vi "Reentrancy String.vi"(7 "Format Options":T1={"Background"={"Public Scope"={"Option"=FALSE, "Color"=0, "Operator"=FALSE}, "Protected Scope"={"Option"=FALSE, "Color"=0, "Operator"=FALSE}, "Community Scope"={"Option"=FALSE, "Color"=0, "Operator"=FALSE}, "Private Scope"={"Option"=FALSE, "Color"=0, "Operator"=FALSE}, "Unknown Scope"={"Option"=FALSE, "Color"=0, "Operator"=FALSE}, "Auto Error Handling"={"Option"=FALSE, "Color"=0, "Operator"=FALSE}, "Inline"={"Option"=FALSE, "Color"=0, "Operator"=FALSE}, "Separate CC"={"Option"=FALSE, "Color"=0, "Operator"=FALSE}, "Execution Priority Normal"={"Option"=FALSE, "Color"=0, "Operator"=FALSE}, "Reentrancy Non-RE"={"Option"=FALSE, "Color"=0, "Operator"=FALSE}}, "Bookmark Options"={"Bookmarks as New Line in VI Descriptions"=TRUE, "Unique Bookmark Tags Only"=TRUE, "Include Tag and Text"=TRUE}}, 9 "Exec.IsReentrant":bool, 11 "Exec.ReentrancyType":T4(ring)) -> (1 "Cell Color":u32, 3 "Reentrancy":string)   [LabVIEW 2023, in "VIDoc Printer.lvlib" / "VIDoc Printer.lvclass"]
doc: "Formats Reentrancy information into a string.\nAlso outputs a color based on the Format Options."
uses:
  VIDoc Printer.lvclass
  Settings/Printer Settings/Formatting Options.ctl
  Settings/Printer Settings/Background Formatting Cluster.ctl
  Settings/Printer Settings/Bookmark Options.ctl
  VIDoc Printer.lvclass/VIDoc Printer.ctl
  Settings/Printer Settings/Printer Settings.lvclass
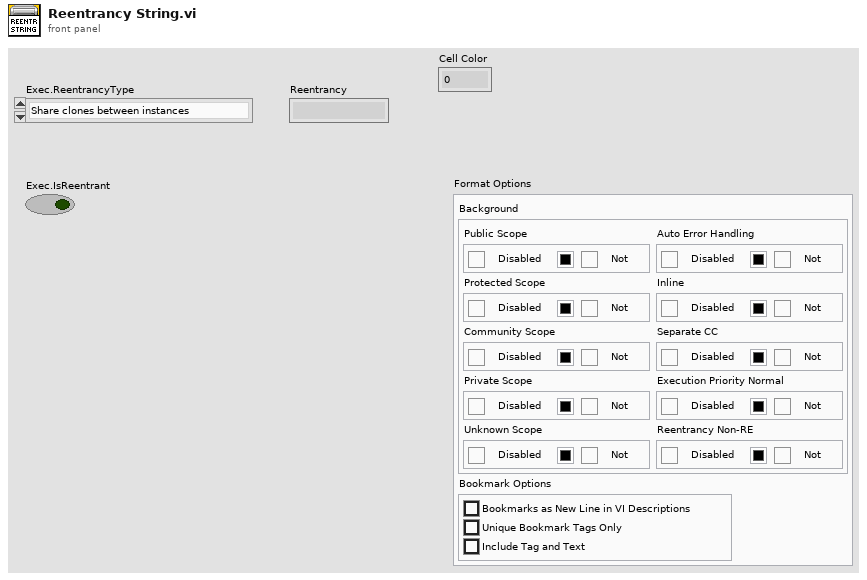
[diagram p1: front panel]
types:
  T1 = typedef "VIDoc Printer.lvlib/Printer Settings.lvclass/Formatting Options.ctl" = cluster{"Background":cluster{"Public Scope":T2, "Protected Scope":T2, "Community Scope":T2, "Private Scope":T2, "Unknown Scope":T2, "Auto Error Handling":T2, "Inline":T2, "Separate CC":T2, "Execution Priority Normal":T2, "Reentrancy Non-RE":T2}, "Bookmark Options":T3}
  T2 = typedef "VIDoc Printer.lvlib/Printer Settings.lvclass/Background Formatting Cluster.ctl" = cluster{"Option":bool, "Color":u32, "Operator":bool}
  T3 = typedef "VIDoc Printer.lvlib/Printer Settings.lvclass/Bookmark Options.ctl" = cluster{"Bookmarks as New Line in VI Descriptions":bool, "Unique Bookmark Tags Only":bool, "Include Tag and Text":bool}
  T4 = enum16{"Share clones between instances", "Preallocate clone for each instance"}
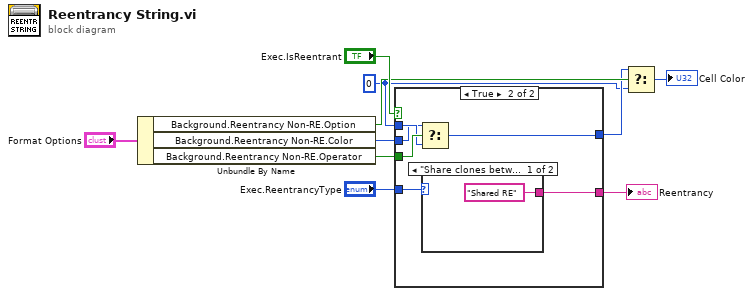
[diagram p0: block diagram]
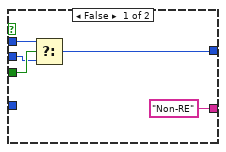
[diagram p2: hidden frame]
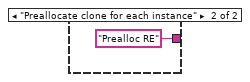
[diagram p3: hidden frame]
diagram:
  w2 = 0
  n1 = Unbundle By Name("Format Options") -> ("Background.Reentrancy Non-RE.Option"=w7:bool, "Background.Reentrancy Non-RE.Color"=w6:u32, "Background.Reentrancy Non-RE.Operator"=w4:bool)
  n2 = case shown="True" "Exec.IsReentrant" {
    tunnel: ["Non-RE" w20] -> w9
    tunnel: "Exec.ReentrancyType" -> [_ w21]
    tunnel: w6 -> [w13 w17]
    tunnel: [w11 w16] -> w5
    tunnel: w4 -> [w14 w19]
    tunnel: w2 -> [w12 w18]
    frame False {
      n3 = Select(t=w12, s=w14, f=w13) -> (s? t:f=w11:u32)
    }
    frame True {
      n4 = Select(t=w17, s=w19, f=w18) -> (s? t:f=w16:u32)
      n5 = case shown="\"Share clones between instances\"" w21 {
        tunnel: ["Shared RE" "Prealloc RE"] -> w20
        frame "Share clones between instances" {
        }
        frame "Preallocate clone for each instance" {
        }
      }
    }
  }
  "Reentrancy" <- w9
  n6 = Select(t=w5, s=w7, f=w2) -> (s? t:f=→"Cell Color":u32)
